vi "Kinect_to_3D.vi"(0 "previous_X_3D":dbl, 1 "current_X_kinect":dbl, 2 "previous_X_kinect":dbl, 3 "previous_Y_3D":dbl, 4 "current_Y_kinect":dbl, 5 "previous_Y_kinect":dbl, 6 "previous_Z_kinect":dbl, 7 "X_Y_speed":dbl, 8 "current_Z_kinect":dbl, 9 "Z_speed":dbl, 10 "previous_Z_3D":dbl) -> (14 "X_3D":dbl, 15 "Y_3D":dbl, 16 "Z_3D":dbl, 17 "Xmax":dbl=2.5, 18 "Ymax":dbl, 19 "Zmax":dbl=2.5)   [LabVIEW 2011]
panel:
  out "X_resolution":i16
  out "Y_resolution":i16
  out "Y_scaling":dbl
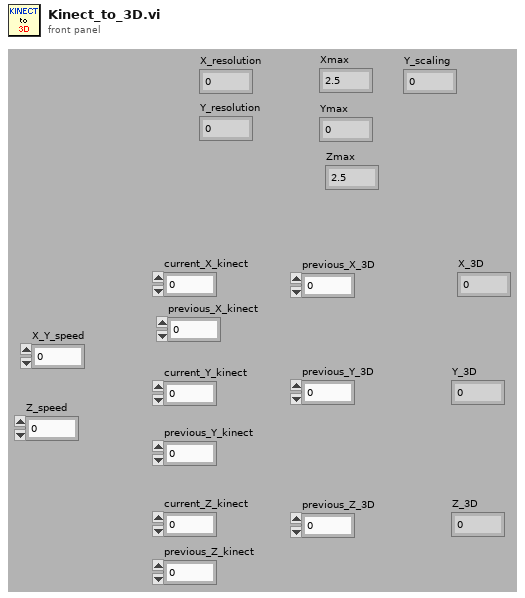
[diagram p1: front panel]
types:
  T1 = typedef "LVAllMonitorsDisplayTypeDef.ctl" = cluster{"Bounds":cluster{"Left":i16, "Top":i16, "Right":i16, "Bottom":i16}, "Depth":i16}[]
  T2 = cluster{"Bounds":cluster{"Left":i16, "Top":i16, "Right":i16, "Bottom":i16}, "Depth":i16}
  T3 = cluster{"Left":i16, "Top":i16, "Right":i16, "Bottom":i16}
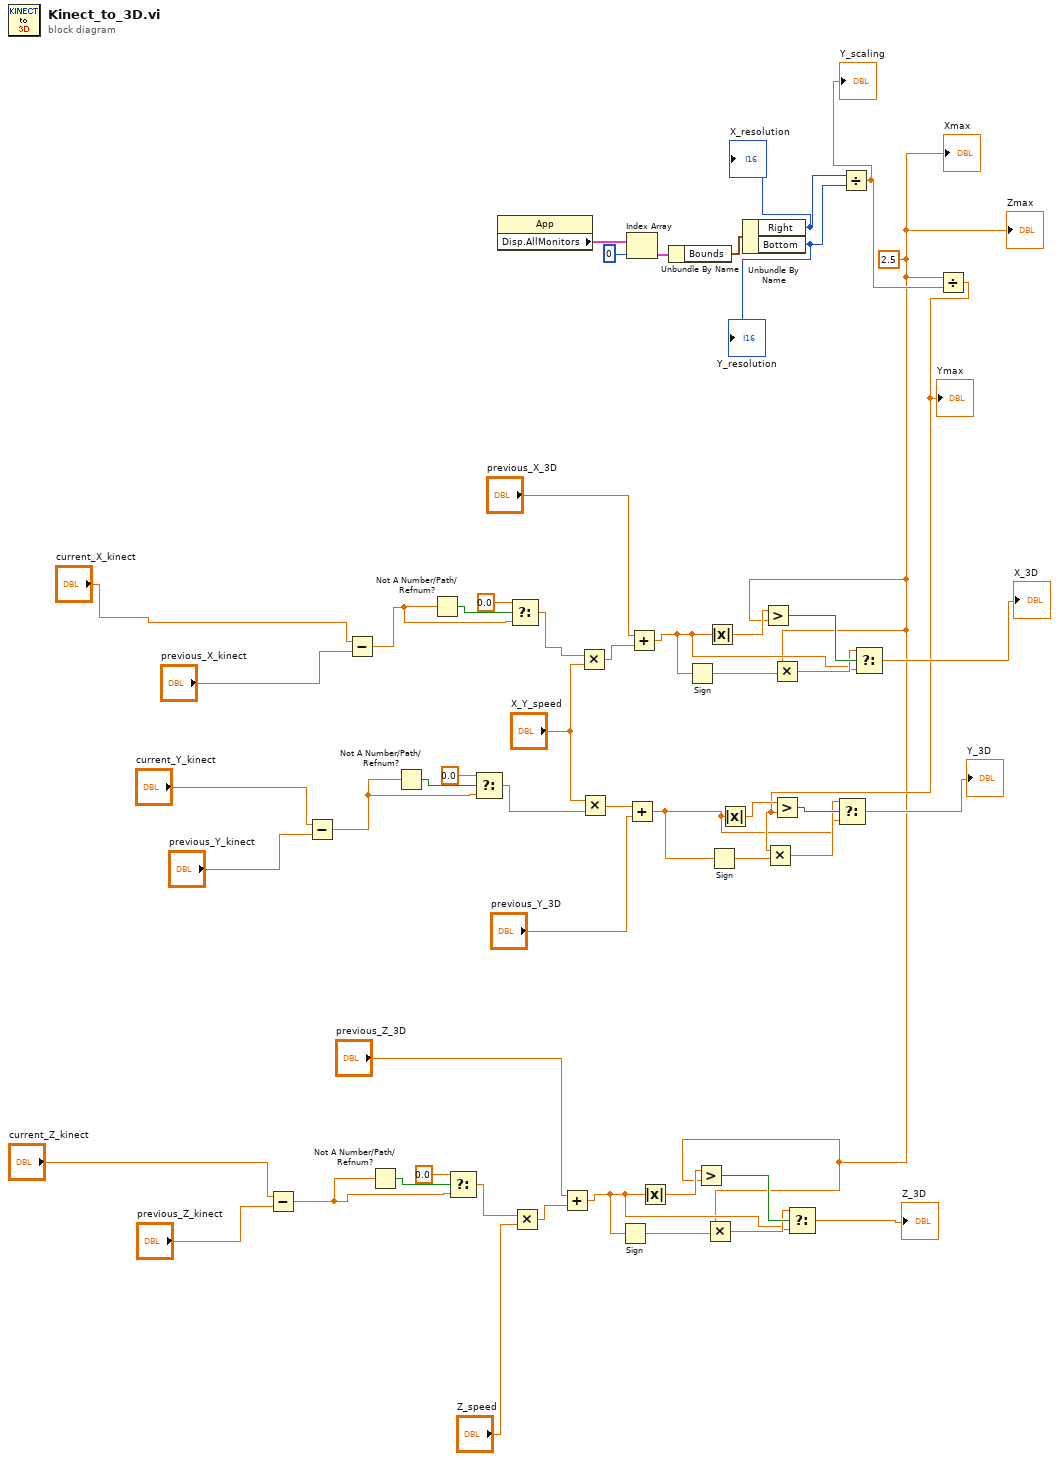
[diagram p0: block diagram]
diagram:
  w21 = 2.5 ("x")
  n1 = Subtract(x="current_Z_kinect", y="previous_Z_kinect") -> (x-y=w2:dbl)
  n2 = Subtract(x="current_Y_kinect", y="previous_Y_kinect") -> (x-y=w8:dbl)
  n3 = Subtract(x="current_X_kinect", y="previous_X_kinect") -> (x-y=w13:dbl)
  n4 = Not A Number/Path/Refnum?(number/path/refnum=w2) -> (NaN/Path/Refnum?=w5:bool)
  n5 = Not A Number/Path/Refnum?(number/path/refnum=w8) -> (NaN/Path/Refnum?=w10:bool)
  n6 = Not A Number/Path/Refnum?(number/path/refnum=w13) -> (NaN/Path/Refnum?=w15:bool)
  n7 = Select(t=0.0, s=w5, f=w2) -> (s? t:f=w3:dbl)
  n8 = Select(t=0.0, s=w10, f=w8) -> (s? t:f=w7:dbl)
  n9 = property class="App"() -> ("Disp.AllMonitors"=w51:T1)  [unwired: 2 in, 2 out]
  n10 = Select(t=0.0, s=w15, f=w13) -> (s? t:f=w12:dbl)
  n11 = Multiply(x=w3, y="Z_speed") -> (x*y=w29:dbl)
  n12 = Add(x="previous_Z_3D", y=w29) -> (x+y=w23:dbl)
  n13 = Multiply(x=w12, y="X_Y_speed") -> (x*y=w46:dbl)
  n14 = Multiply(x="X_Y_speed", y=w7) -> (x*y=w44:dbl)
  n15 = Sign(1:w23) -> (0:w25:dbl)
  n16 = Index Array(array=w51, index=u16 0 ("Front Panel Window:Monitor")) -> (element=w53:T2)
  n17 = Add(x=w44, y="previous_Y_3D") -> (x+y=w31:dbl)
  n18 = Add(x="previous_X_3D", y=w46) -> (x+y=w37:dbl)
  n19 = Absolute Value(x=w23) -> (abs(x)=w27:dbl)
  n20 = Unbundle By Name(w53) -> ("Bounds"=w50:T3)
  n21 = Sign(1:w37) -> (0:w40:dbl)
  n22 = Greater?(x=w27, y=w21) -> (0:w26:bool)
  n23 = Multiply(x=w21, y=w25) -> (x*y=w24:dbl)
  n24 = Absolute Value(x=w37) -> (abs(x)=w42:dbl)
  n25 = Sign(1:w31) -> (0:w33:dbl)
  n26 = Absolute Value(x=w31) -> (abs(x)=w36:dbl)
  n27 = Unbundle By Name(w50) -> ("Right"=w48:i16, "Bottom"=w49:i16)
  "Y_resolution" <- w49
  "X_resolution" <- w48
  n28 = Greater?(x=w42, y=w21) -> (0:w41:bool)
  n29 = Multiply(x=w21, y=w40) -> (x*y=w39:dbl)
  n30 = Select(t=w24, s=w26, f=w23) -> (s? t:f=→"Z_3D":dbl)
  n31 = Divide(x=w48, y=w49) -> (x/y=w47:dbl)
  "Y_scaling" <- w47
  n32 = Select(t=w39, s=w41, f=w37) -> (s? t:f=→"X_3D":dbl)
  n33 = Divide(x=w21, y=w47) -> (x/y=w34:dbl)
  "Ymax" <- w34
  n34 = Multiply(x=w34, y=w33) -> (x*y=w32:dbl)
  n35 = Greater?(x=w36, y=w34) -> (0:w35:bool)
  n36 = Select(t=w32, s=w35, f=w31) -> (s? t:f=→"Y_3D":dbl)
  "Xmax" <- w21
  "Zmax" <- w21
